vi "RasterScan.vi"(0 "Optical Input":T1, 1 "Optical Output":T2, 2 "Stage Port":refnum<visa-resource-name>, 3 "x-axis stage":string, 4 "y-axis stage":string, 5 "error in (no error)":errorcluster, 6 "Detectors Select":enum32{"4 Detectors", "8 Detectors"}(ring), 7 "DAQ Port":tag, 8 "X Steps":i32, 9 "Detector Buttons":refnum<vi>, 10 "Y Steps":i32, 11 "Detector Indicator":refnum<vi>, 12 "Microstep resolution":dbl, 13 "Time Left (ms)":refnum<vi>, 14 "X Increment [mm]":dbl, 15 "Update Time (ms):":refnum<vi>, 16 "Y Increment [mm]":dbl, 17 "Duration Time (ms):":refnum<vi>, 18 "x index":refnum<vi>, 19 "Computer time":refnum<vi>, 20 "y index":refnum<vi>, 21 "File Path:":path, 22 "File Name:":string, 25 "Raster X Reverse":bool, 26 "g2":refnum<vi>, 27 "Position array":refnum<vi>[](array[refnum])) -> (23 "VISA Refnum out":refnum<visa-resource-name>, 24 "error out":errorcluster)   [LabVIEW 2011]
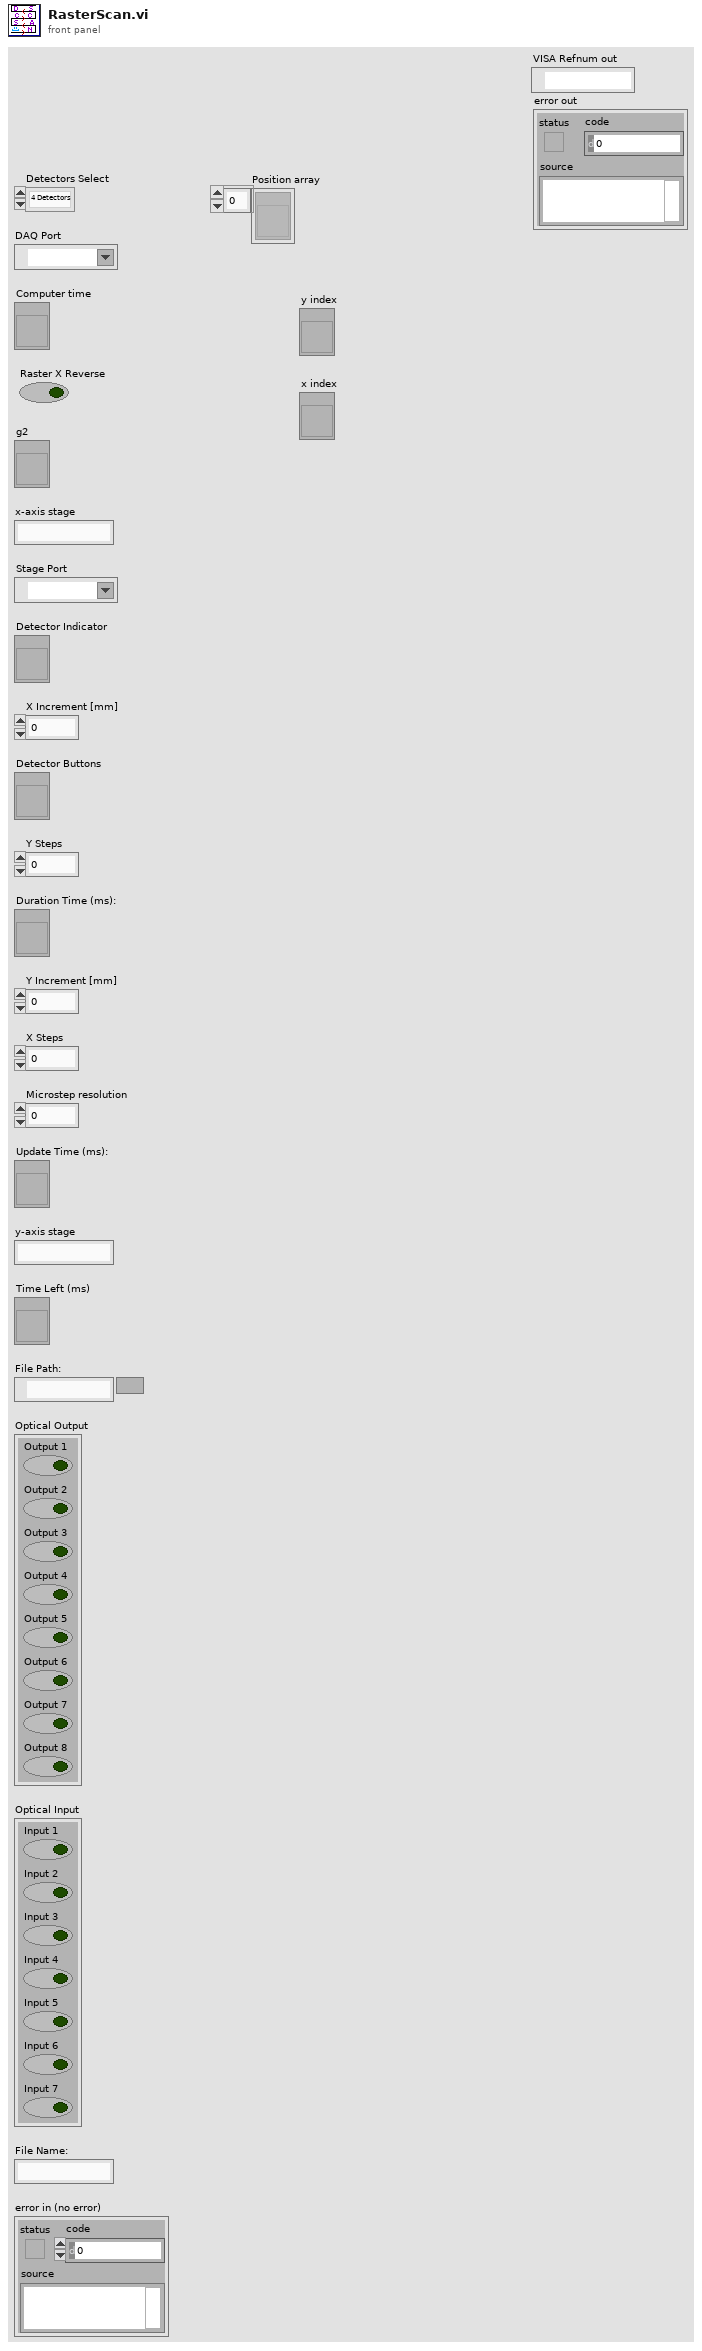
[diagram p1: front panel]
types:
  T1 = cluster{"Input 1":bool, "Input 2":bool, "Input 3":bool, "Input 4":bool, "Input 5":bool, "Input 6":bool, "Input 7":bool}
  T2 = cluster{"Output 1":bool, "Output 2":bool, "Output 3":bool, "Output 4":bool, "Output 5":bool, "Output 6":bool, "Output 7":bool, "Output 8":bool}
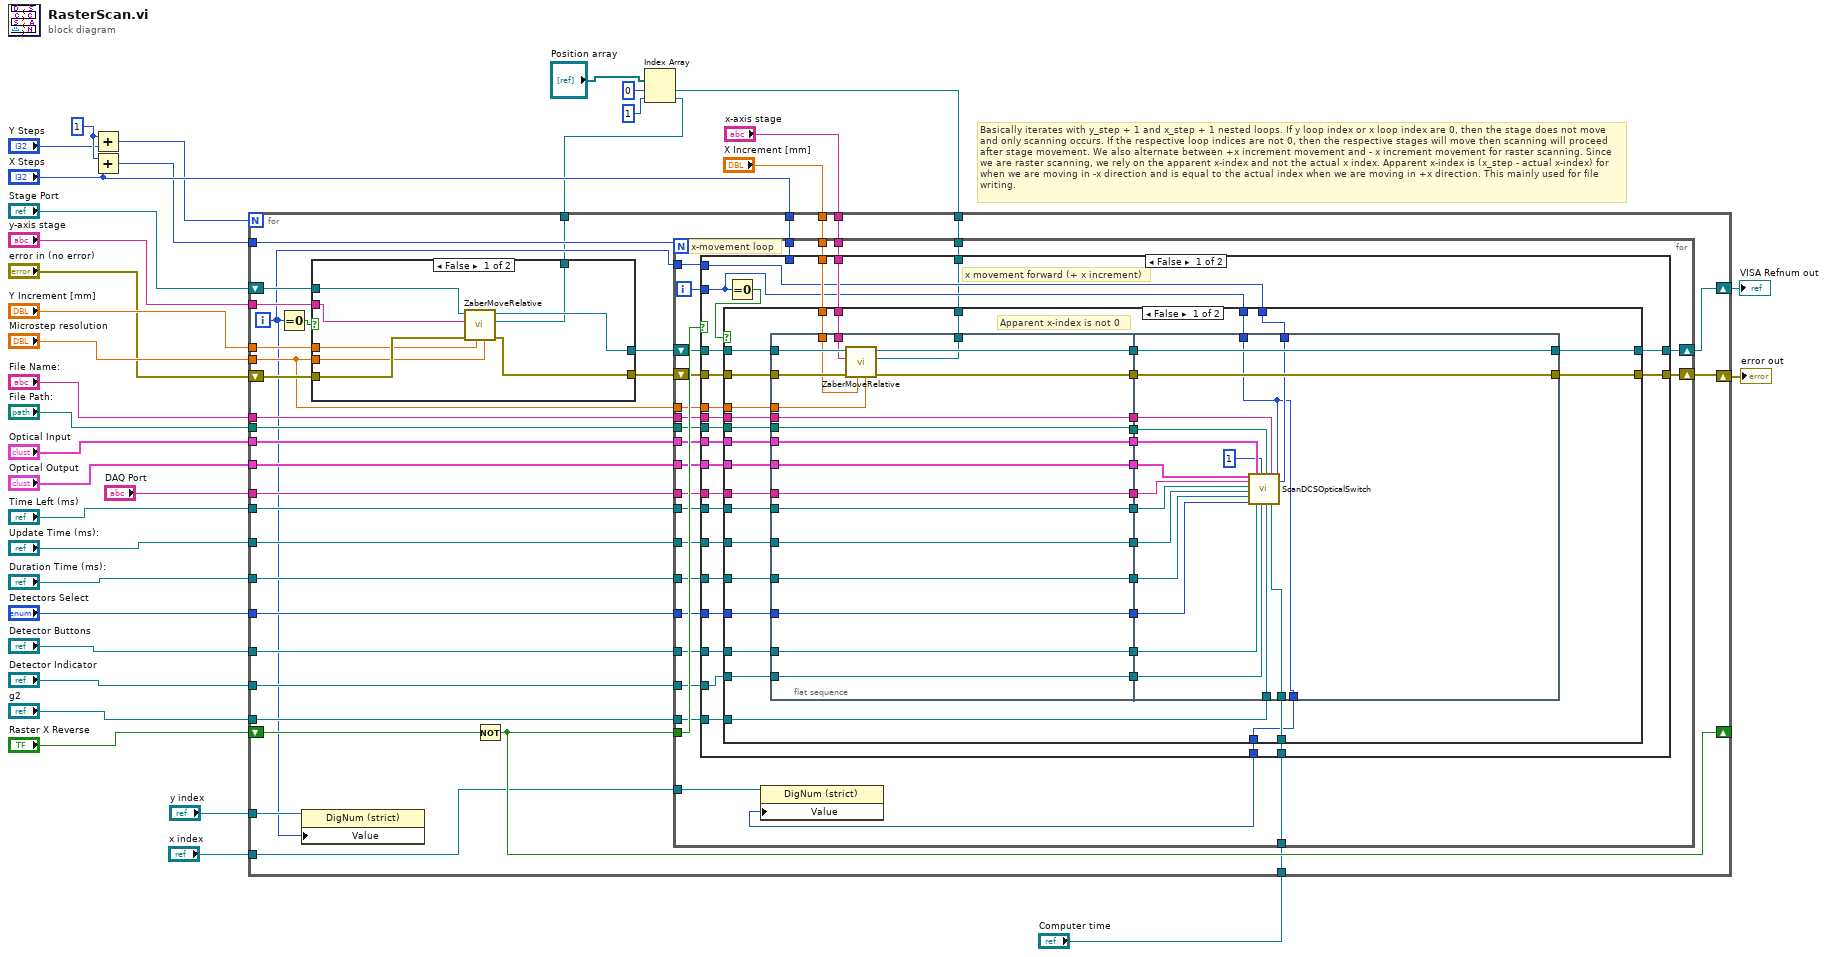
[diagram p0: block diagram]
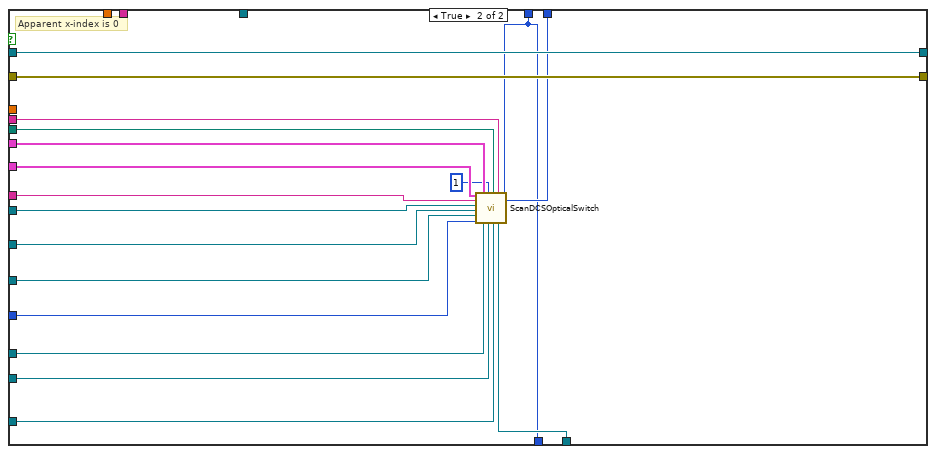
[diagram p3: hidden frame]
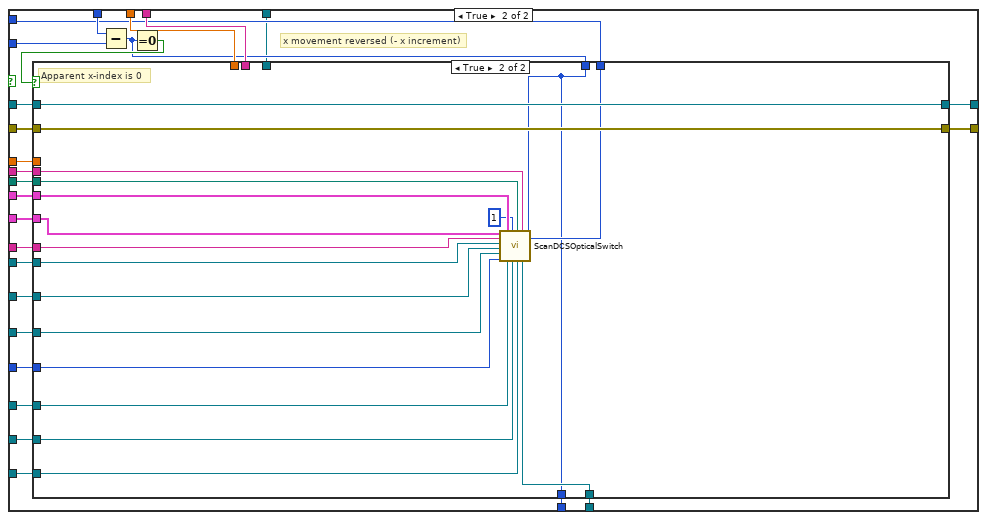
[diagram p4: hidden frame]
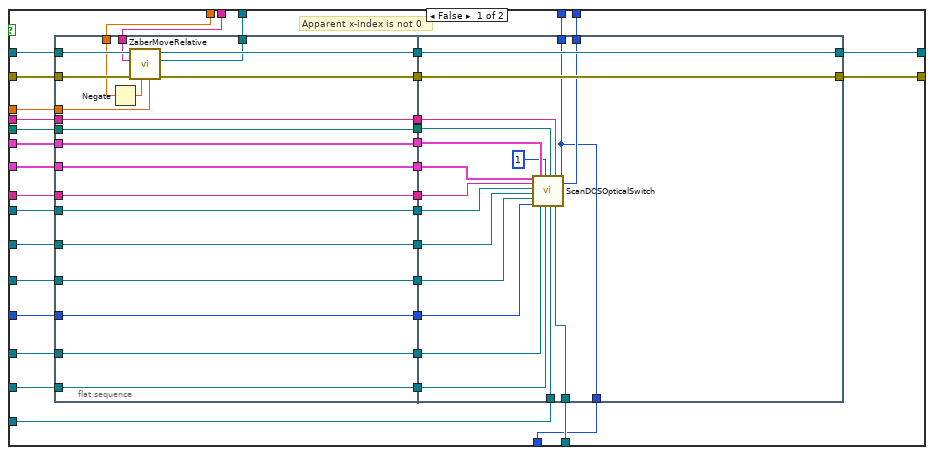
[diagram p5: hidden frame]
diagram:
  w11 = 1
  # "Basically iterates with y_step + 1 and x_step + 1 nested loops. If y loop index or x loop index are 0, then the stage does not move and only scanning occurs. If the respective loop indices are not 0, then the respective stages will move then scanning will proceed after stage movement. We also alternate between +x increment movement and - x increment movement for raster scanning. Since we are raster scanning, we rely on the apparent x-index and not the actual x index. Apparent x-index is (x_step - actual x-index) for when we are moving in -x direction and is equal to the actual index when we are moving in +x direction. This mainly used for file writing."
  n1 = Add(x=w11, y="Y Steps") -> (x+y=w12:i32)
  n2 = Add(x=w11, y="X Steps") -> (x+y=w13:i32)
  n3 = Index Array(array="Position array", index #1=0, index #2=1) -> (element #1=w2:refnum<vi>, element #2=w1:refnum<vi>)
  n4 = for {
    N: w12 -> [_]
    tunnel: w13 -> [w66]
    shift-right: [w67] -> _
    shift-left: "Raster X Reverse" -> [w68]
    tunnel: "Detectors Select" -> [w65]
    tunnel: "Duration Time (ms):" -> [w64]
    tunnel: "Update Time (ms):" -> [w63]
    tunnel: "Time Left (ms)" -> [w62]
    tunnel: "Detector Buttons" -> [w61]
    tunnel: "Detector Indicator" -> [w60]
    tunnel: "g2" -> [w59]
    tunnel: "y-axis stage" -> [w56]
    tunnel: "Y Increment [mm]" -> [w55]
    tunnel: "Microstep resolution" -> [w49]
    tunnel: "x-axis stage" -> [w52]
    shift-right: [w51] -> w9
    shift-left: "Stage Port" -> [w58]
    shift-right: [w50] -> w8
    shift-left: "error in (no error)" -> [w57]
    tunnel: "X Increment [mm]" -> [w48]
    tunnel: "X Steps" -> [w47]
    tunnel: "Optical Input" -> [w46]
    tunnel: "Optical Output" -> [w45]
    tunnel: "Computer time" -> [w44]
    tunnel: "DAQ Port" -> [w43]
    tunnel: "File Name:" -> [w42]
    tunnel: "File Path:" -> [w41]
    tunnel: "y index" -> [w40]
    tunnel: "x index" -> [w38]
    tunnel: w2 -> [w37]
    tunnel: w1 -> [w36]
    i -> [w39]
    n5 = Equal To 0?(x=w39) -> (x = 0?=w69:bool)
    n6 = property class="DigNum (strict)"(reference=w40, "Value"=w39) -> ()  [unwired: 1 in, 2 out]
    n7 = case shown="False" w69 {
      tunnel: w58 -> [w77 w79]
      tunnel: w57 -> [w76 w78]
      tunnel: w56 -> [w75 _]
      tunnel: w55 -> [w74 _]
      tunnel: w49 -> [w73 _]
      tunnel: [w72 w79] -> w54
      tunnel: [w71 w78] -> w53
      tunnel: w36 -> [w70 _]
      frame False {
        n8 = call "ZaberMoveRelative.vi"("Position Indicator"=w70, "Microstep resolution"=w73, "distance [mm]"=w74, "error in (no error)"=w76, "Device"=w75, "VISA Refnum in"=w77) -> ("error out"=w71:errorcluster, "VISA Refnum out"=w72:refnum<visa-resource-name>)  [unwired: 4 in]
      }
      frame True {
      }
    }
    n9 = Not(x=w68) -> (.not. x?=w67:bool)
    n10 = for {
      N: w66 -> [_]
      tunnel: w67 -> [w106]
      tunnel: w65 -> [w105]
      tunnel: w64 -> [w104]
      tunnel: w63 -> [w103]
      tunnel: w62 -> [w102]
      tunnel: w61 -> [w101]
      tunnel: w60 -> [w100]
      tunnel: w59 -> [w99]
      tunnel: w46 -> [w98]
      tunnel: w45 -> [w97]
      tunnel: w52 -> [w94]
      shift-right: [w93] -> w51
      shift-left: w54 -> [w96]
      shift-right: [w92] -> w50
      shift-left: w53 -> [w95]
      tunnel: w49 -> [w91]
      tunnel: w48 -> [w90]
      tunnel: w47 -> [w89]
      tunnel: w44 -> [w88]
      tunnel: w43 -> [w87]
      tunnel: w42 -> [w86]
      tunnel: w41 -> [w85]
      tunnel: w39 -> [w84]
      tunnel: w38 -> [w83]
      tunnel: w37 -> [w80]
      i -> [w82]
      # "x-movement loop"
      n11 = case shown="False" w106 {
        tunnel: w82 -> [w110 w250]
        tunnel: w105 -> [w119 w248]
        tunnel: w104 -> [w118 w247]
        tunnel: w103 -> [w117 w246]
        tunnel: w102 -> [w116 w245]
        tunnel: w101 -> [w120 w244]
        tunnel: w100 -> [w121 w243]
        tunnel: w99 -> [w122 w242]
        tunnel: w98 -> [w113 w241]
        tunnel: w97 -> [w114 w240]
        tunnel: w96 -> [w130 w237]
        tunnel: w95 -> [w129 w236]
        tunnel: w94 -> [w128 w239]
        tunnel: [w127 w227] -> w93
        tunnel: [w126 w226] -> w92
        tunnel: w91 -> [w125 w235]
        tunnel: w90 -> [w124 w238]
        tunnel: w89 -> [_ w234]
        tunnel: w88 -> [w123 w233]
        tunnel: w87 -> [w115 w232]
        tunnel: w86 -> [w112 w230]
        tunnel: w85 -> [w111 w231]
        tunnel: w84 -> [w109 w228]
        tunnel: [w108 w225] -> w81
        tunnel: w80 -> [w107 w224]
        frame False {
          # "x movement forward (+ x increment)"
          n12 = Equal To 0?(x=w110) -> (x = 0?=w131:bool)
          n13 = case shown="False" w131 {
            tunnel: w130 -> [w168 w223]
            tunnel: w129 -> [w167 w222]
            tunnel: w128 -> [w166 _]
            tunnel: [w163 w223] -> w127
            tunnel: [w162 w222] -> w126
            tunnel: w125 -> [w161 _]
            tunnel: w124 -> [w160 _]
            tunnel: w123 -> [w159 w221]
            tunnel: w122 -> [w158 w220]
            tunnel: w121 -> [w156 w219]
            tunnel: w120 -> [w154 w218]
            tunnel: w119 -> [w152 w217]
            tunnel: w118 -> [w150 w216]
            tunnel: w117 -> [w148 w215]
            tunnel: w116 -> [w146 w214]
            tunnel: w115 -> [w144 w213]
            tunnel: w114 -> [w142 w212]
            tunnel: w113 -> [w141 w211]
            tunnel: w112 -> [w138 w209]
            tunnel: w111 -> [w136 w210]
            tunnel: w110 -> [w135 w206]
            tunnel: w109 -> [w134 w208]
            tunnel: [w133 w206] -> w108
            tunnel: w107 -> [w132 _]
            frame False {
              # "Apparent x-index is not 0"
              n14 = flat-sequence {
                tunnel: w168 -> [w187]
                tunnel: w167 -> [w186]
                tunnel: w166 -> [w185]
                tunnel: [w184] -> w165
                tunnel: [w183] -> w164
                tunnel: w161 -> [w182]
                tunnel: w160 -> [w170]
                tunnel: [w181] -> w157
                tunnel: w156 -> [w181]
                tunnel: [w180] -> w155
                tunnel: w154 -> [w180]
                tunnel: [w179] -> w153
                tunnel: w152 -> [w179]
                tunnel: [w178] -> w151
                tunnel: w150 -> [w178]
                tunnel: [w177] -> w149
                tunnel: w148 -> [w177]
                tunnel: [w176] -> w147
                tunnel: w146 -> [w176]
                tunnel: [w175] -> w145
                tunnel: w144 -> [w175]
                tunnel: [w174] -> w143
                tunnel: w142 -> [w174]
                tunnel: w141 -> [w173]
                tunnel: [w173] -> w140
                tunnel: [w172] -> w139
                tunnel: w138 -> [w172]
                tunnel: [w171] -> w137
                tunnel: w136 -> [w171]
                tunnel: w132 -> [w169]
                tunnel: [w205] -> w163
                tunnel: w165 -> [w205]
                tunnel: [w204] -> w162
                tunnel: w164 -> [w204]
                tunnel: w159 -> [w203]
                tunnel: w158 -> [w202]
                tunnel: w157 -> [w201]
                tunnel: w155 -> [w200]
                tunnel: w153 -> [w199]
                tunnel: w151 -> [w198]
                tunnel: w149 -> [w197]
                tunnel: w147 -> [w196]
                tunnel: w145 -> [w195]
                tunnel: w143 -> [w194]
                tunnel: w140 -> [w193]
                tunnel: w139 -> [w192]
                tunnel: w137 -> [w191]
                tunnel: w135 -> [w188]
                tunnel: w134 -> [w189]
                tunnel: [w188] -> w133
                frame #0 {
                  n15 = call "ZaberMoveRelative.vi"("Position Indicator"=w169, "Microstep resolution"=w182, "distance [mm]"=w170, "error in (no error)"=w186, "Device"=w185, "VISA Refnum in"=w187) -> ("error out"=w183:errorcluster, "VISA Refnum out"=w184:refnum<visa-resource-name>)  [unwired: 4 in]
                }
                frame #1 {
                  n16 = call "ScanDCSOpticalSwitch.vi"("Optical Output"=w194, "DAQ Port"=w195, "Time Left (ms)"=w196, "Update Time (ms):"=w197, "Duration Time (ms):"=w198, "Detectors Select"=w199, "Optical Input"=w193, "Detector\n Buttons"=w200, "Number of Scans"=1, "Detector Indicator"=w201, "File Path:"=w191, "g2"=w202, "File Name:"=w192, "Computer time"=w203, "X index"=w188, "Y index"=w189) -> ()  [unwired: 4 in]
                }
              }
            }
            frame True {
              # "Apparent x-index is 0"
              n17 = call "ScanDCSOpticalSwitch.vi"("Optical Output"=w212, "DAQ Port"=w213, "Time Left (ms)"=w214, "Update Time (ms):"=w215, "Duration Time (ms):"=w216, "Detectors Select"=w217, "Optical Input"=w211, "Detector\n Buttons"=w218, "Number of Scans"=1, "Detector Indicator"=w219, "File Path:"=w210, "g2"=w220, "File Name:"=w209, "Computer time"=w221, "X index"=w206, "Y index"=w208) -> ()  [unwired: 4 in]
            }
          }
        }
        frame True {
          # "x movement reversed (- x increment)"
          n18 = Subtract(x=w234, y=w250) -> (x-y=w229:i32)
          n19 = Equal To 0?(x=w229) -> (x = 0?=w249:bool)
          n20 = case shown="True" w249 {
            tunnel: w248 -> [w273 w337]
            tunnel: w247 -> [w271 w336]
            tunnel: w246 -> [w269 w335]
            tunnel: w245 -> [w267 w334]
            tunnel: w244 -> [w276 w338]
            tunnel: w243 -> [w278 w339]
            tunnel: w242 -> [w279 w340]
            tunnel: w241 -> [w261 w331]
            tunnel: w240 -> [w263 w332]
            tunnel: w239 -> [w284 _]
            tunnel: w238 -> [w285 _]
            tunnel: w237 -> [w283 w343]
            tunnel: w236 -> [w282 w342]
            tunnel: w235 -> [w281 _]
            tunnel: w233 -> [w280 w341]
            tunnel: w232 -> [w265 w333]
            tunnel: w231 -> [w259 w330]
            tunnel: w230 -> [w258 w329]
            tunnel: w229 -> [w256 w326]
            tunnel: w228 -> [w255 w328]
            tunnel: [w254 w343] -> w227
            tunnel: [w253 w342] -> w226
            tunnel: [w252 w326] -> w225
            tunnel: w224 -> [w251 _]
            frame False {
              # "Apparent x-index is not 0"
              n21 = flat-sequence {
                tunnel: w283 -> [w307]
                tunnel: w282 -> [w306]
                tunnel: w284 -> [w305]
                tunnel: [w304] -> w287
                tunnel: [w303] -> w286
                tunnel: w281 -> [w302]
                tunnel: w285 -> [w289]
                tunnel: w278 -> [w301]
                tunnel: [w301] -> w277
                tunnel: w276 -> [w300]
                tunnel: [w300] -> w275
                tunnel: [w299] -> w274
                tunnel: w273 -> [w299]
                tunnel: [w298] -> w272
                tunnel: w271 -> [w298]
                tunnel: [w297] -> w270
                tunnel: w269 -> [w297]
                tunnel: [w296] -> w268
                tunnel: w267 -> [w296]
                tunnel: [w295] -> w266
                tunnel: w265 -> [w295]
                tunnel: [w294] -> w264
                tunnel: w263 -> [w294]
                tunnel: [w293] -> w262
                tunnel: w261 -> [w293]
                tunnel: [w292] -> w260
                tunnel: w259 -> [w292]
                tunnel: w258 -> [w291]
                tunnel: [w291] -> w257
                tunnel: w251 -> [w288]
                tunnel: [w325] -> w254
                tunnel: w287 -> [w325]
                tunnel: [w324] -> w253
                tunnel: w286 -> [w324]
                tunnel: w280 -> [w323]
                tunnel: w279 -> [w322]
                tunnel: w277 -> [w321]
                tunnel: w275 -> [w320]
                tunnel: w274 -> [w319]
                tunnel: w272 -> [w318]
                tunnel: w270 -> [w317]
                tunnel: w268 -> [w316]
                tunnel: w266 -> [w315]
                tunnel: w264 -> [w314]
                tunnel: w262 -> [w313]
                tunnel: w260 -> [w312]
                tunnel: w257 -> [w311]
                tunnel: w256 -> [w308]
                tunnel: w255 -> [w310]
                tunnel: [w308] -> w252
                frame #0 {
                  n22 = Negate(x=w289) -> (-x=w290:dbl)
                  n23 = call "ZaberMoveRelative.vi"("Position Indicator"=w288, "Microstep resolution"=w302, "distance [mm]"=w290, "error in (no error)"=w306, "Device"=w305, "VISA Refnum in"=w307) -> ("error out"=w303:errorcluster, "VISA Refnum out"=w304:refnum<visa-resource-name>)  [unwired: 4 in]
                }
                frame #1 {
                  n24 = call "ScanDCSOpticalSwitch.vi"("Optical Output"=w314, "DAQ Port"=w315, "Time Left (ms)"=w316, "Update Time (ms):"=w317, "Duration Time (ms):"=w318, "Detectors Select"=w319, "Optical Input"=w313, "Detector\n Buttons"=w320, "Number of Scans"=1, "Detector Indicator"=w321, "File Path:"=w312, "g2"=w322, "File Name:"=w311, "Computer time"=w323, "X index"=w308, "Y index"=w310) -> ()  [unwired: 4 in]
                }
              }
            }
            frame True {
              # "Apparent x-index is 0"
              n25 = call "ScanDCSOpticalSwitch.vi"("Optical Output"=w332, "DAQ Port"=w333, "Time Left (ms)"=w334, "Update Time (ms):"=w335, "Duration Time (ms):"=w336, "Detectors Select"=w337, "Optical Input"=w331, "Detector\n Buttons"=w338, "Number of Scans"=1, "Detector Indicator"=w339, "File Path:"=w330, "g2"=w340, "File Name:"=w329, "Computer time"=w341, "X index"=w326, "Y index"=w328) -> ()  [unwired: 4 in]
            }
          }
        }
      }
      n26 = property class="DigNum (strict)"(reference=w83, "Value"=w81) -> ()  [unwired: 1 in, 2 out]
    }
  }
  "VISA Refnum out" <- w9
  "error out" <- w8
